vi "声音识别.vi"() -> ()   [LabVIEW 2014]
uses:
  <vilib>/sound/lvsound.llb/Sound Format.ctl
  <vilib>/Analysis/4window.llb/windowTd.ctl
  <vilib>/Analysis/1siggen.llb/Ramp Pattern by Samples.vi
  <vilib>/Analysis/NI_AALPro.lvlib
  <vilib>/Analysis/NI_AALBase.lvlib
panel:
  in  "停止":bool
  out "主频":i32
  in  "低频点":i32=90
  in  "高频点":i32=120
  out "模板2匹配":bool[](array[boolean])
  out "模板1匹配":bool[](array[boolean])
  in  "选项卡控件":enum32{"参数设置", "声卡设置"}(tab)
  in  "存模板1":bool caption="模板1"
  in  "存模板2":bool caption="模板2"
  in  "滤波器类型":i32(ring)=1 items=["低通", "高通", "带通", "带阻"]
  in  "高截止频率":dbl=2000.0 format="%.2f"
  in  "低截止频率":dbl=60.0 format="%.2f"
  in  "阶数":dbl=2.0 format="%.2f"
  in  "滤波器选择":u16(ring) items=["切比雪夫", "巴特沃斯", "无"]
  in  "截取声音长度":u16(ring)=512 items=["256"=256, "512"=512, "1024"=1024, "2048"=2048]
  in  "sound format":T1={"sound quality"=enum."mono", "rate"=enum."44100", "bits per sample"=enum."16 bit"} caption="声音格式"
  out "模板2":dbl[](array[numeric])=[-1.0, -0.9999784757638632, -0.999883730923308, -0.9997268308186364, -0.9996087454137307, -0.9995485640574947, -0.9996660148873113, -0.9996460865374096, -0.9990520630289842, -0.9996447767562398, -0.9988842018427372, -0.9988326168901588, -0.9994362746882363, -0.9994043225637047, -0.9996462893274354, -0.999250094691715, -0.9996529817000758, -0.9990974819147969, -0.9998535553541484, -0.9991407864070688, -0.9996794207758661, -0.9998567670842584, -0.9987714624308643, -0.9988979613875477, -0.9981546271077171, -0.99883165401242, -0.999806679939325, -0.9987834495902463, -0.9987170240934524, -0.9986010051790879, -0.9987859779624924, -0.99882513551929, -0.997846064915957, -0.9984471292033844, -0.9989846697345478, -0.9955902561514854, -0.9969375334942442, -0.9985341827269754, -0.9965219910541883, -0.997115233753815, -0.993177621304976, -0.9965369004229736, -0.996247289114047, -0.9965205723109544, -0.9929438024310587, -0.9921813234142332, -0.9923201356826735, -0.9902234197893732, -0.9875050624228046, -0.989978196297217, -0.9899613444021288, -0.9918200276943172, -0.9971748873436627, -0.9936090106840292, -0.9967077448120892, -0.99511317548537, -0.9900547089248353, -0.9915800418719736, -0.9951413205793777, -0.9983222383099732, -0.9983608025847126, -0.9943812759685029, -0.9907756695115925, -0.9910720617475026, -0.9942178283545733, -0.9960071684133079, -0.9947937292245801, -0.9894896646443787, -0.9936749087846007, -0.9986512039031801, -0.9924143125896042, -0.980352872634244, -0.9824158782190716, -0.9882635976611835, -0.9901615400254588, -0.9919879388627098, -0.9929695103692736, -0.9877372544473346, -0.9805321538200102, -0.9723162365341282, -0.9941849154146257, -0.9840418140212489, -0.9785614847877063, -0.9824280510357281, -0.9867776675701149, -0.989155265948291, -0.959160539004141, -0.9312115293907393, -0.924354536297946, -0.9169346034235589, -0.8821247424630705, -0.8638200718968311, -0.8820381048063836, -0.8904287781253226, -0.9186931656047802, -0.942467209539949, -0.9699323519669453, -0.9250753283046158, -0.8718873253555477, -0.8098010457230395, -0.6438727171847084, -0.5912443735241202, -0.7180949540210455, -0.7925349074727238, -0.8919213441425387, -0.8216144716655984, -0.5368039369940907, 0.38886068201338786, 1.0, 0.6065901128787996, -0.20578452524169594, -0.7248999522627186, -0.2749060806920392, 0.07040699283848677, 0.20626459396102206, -0.6102790238762816, -0.9134055836786642, -0.7114504523727746, -0.7787453756820504, -0.859195534470781, -0.6880456234367622, -0.7299328777920452, -0.8034112990123619, -0.7055433624855977, -0.6209224724888913, -0.6474430060007278, -0.6853656731838219, -0.7880905992092426, -0.7444394149310075, -0.9645654801987125, -0.7999452801476307, -0.752200101981826, -0.8948902768790076, -0.8933806119480991, -0.8823017299687642, -0.890886560515635, -0.8894321070807407, -0.8931547753090853, -0.9024438478576883, -0.9100495728196057, -0.911710889209407, -0.9445607561993957, -0.934249135253627, -0.904622091171806, -0.9145055185111371, -0.9628988334908968, -0.9810482464122726, -0.9675874443472068, -0.9621073803076765, -0.9713548954675296, -0.9660622852612207, -0.9439683935237438, -0.9418754698265419, -0.8686568800086364, -0.8092213616083905, -0.940425733399551, -0.9776850827528062, -0.8862970504440179, -0.9269686448441248, -0.9099397807879568, -0.871091321004459, -0.9251669503520498, -0.870146078274874, -0.8803470041783565, -0.6713148081403661, -0.5631453856847152, -0.7665886339386746, -0.9281502818635933, -0.8585161842069289, -0.8024715744018525, -0.8640915179082923, -0.982903824511303, -0.9084909144977602, -0.9722706899843834, -0.9511848674781466, -0.9756589379575122, -0.9787725658314163, -0.9779327416650971, -0.9439377043809586, -0.9291086359847139, -0.8921828883844908, -0.9143793651663683, -0.9233756179572645, -0.9185923843915021, -0.9318259983275918, -0.9312581662523354, -0.8123630832803784, -0.9058753941243535, -0.9432787247324338, -0.9211728624213069, -0.9207238178928795, -0.9020317894743983, -0.8030669530300928, -0.9149433950504898, -0.8616148769398828, -0.7970254148485149, -0.8422440070070124, -0.9125984117938313, -0.9666901859057956, -0.9554246868812509, -0.9894087763072112, -0.956459144652997, -0.9895936405317033, -0.9508371758791279, -0.9200188029869003, -0.9188388870802612, -0.9054584481957318, -0.9429600768930849, -0.9565453895181422, -0.912122419053691, -0.9518819229936425, -0.932683087820026, -0.9278028819493312, -0.9301165652301076, -0.9884957237600749, -0.963040376268851, -0.9655209194019106, -0.8980835146551925, -0.9071915985495637, -0.9562287296834957, -0.9291749404704612, -0.9502166274672502, -0.9843686847549361, -0.9582630331876297, -0.8514277714051874, -0.7171092057916761, -0.8531934139857488, -0.8057421106827759, -0.8013364169222371, -0.9706880418566048, -0.8994513795348863, -0.9430807290280687, -0.9803151690247353, -0.9414492030738784, -0.904749386470448, -0.8410294328838792, -0.8592362276422876, -0.8980549109925963, -0.9065637180637752, -0.9723695887006282, -0.8340799186010609, -0.8754020273712404, -0.940559734933539, -0.9521721965413019, -0.9548370301034873, -0.9603664110042679, -0.9433150050402023, -0.9925992527688022, -0.9720221075238545, -0.9797270980151095, -0.9706349822484007, -0.9919448347863793, -0.9852729642178658, -0.9949885259257842, -0.9770438736058363, -0.9700011832631854]
  out "模板1":dbl[](array[numeric])=[-0.9997440127807419, -0.9995220380571057, -0.9995902897348935, -0.9995357979586109, -0.9994879869517296, -0.9990814431600478, -0.999786870970356, -0.9991893733117945, -0.9998465713309023, -0.9998707870681628, -0.9999563774756277, -0.9983672987139602, -0.999880264902219, -0.9993717852254479, -0.9991030261051548, -0.9995136326835645, -0.9997645347029909, -0.9985313282076574, -0.9997301559393635, -0.9995234641757678, -0.9996431234057226, -0.999139315259616, -0.9995276217859526, -0.9991242785698715, -0.9991479330256554, -0.9992196130388197, -0.9978959279716081, -0.9995639207224252, -0.9985822974140731, -0.9960125349611552, -0.9980838017535006, -0.9964893672759322, -0.9946562731730431, -0.9969521384471256, -0.9959308295729385, -0.9957103403740175, -0.9966716950068587, -0.9969435987481197, -0.9967517577400672, -0.9934997828913328, -0.9952175081092053, -0.9984728596833808, -0.9983665702302467, -0.9953053980437071, -0.9899940068948201, -0.9927011727038199, -0.9974143037244904, -0.9920868374069218, -0.9915651780543104, -0.9946819848753914, -0.9902623232266299, -0.9923224250688908, -0.9962090994146557, -0.9974990188187914, -0.9987799073938248, -0.9964858261875376, -1.0, -0.9950122965483968, -0.9929111542282759, -0.99674771208652, -0.9954380057482245, -0.9960183527965598, -0.9932474770197688, -0.9924202965886824, -0.9937159036114802, -0.9961277720648933, -0.994216636633258, -0.9875978417778765, -0.9882092513484788, -0.9949915495928041, -0.9955829244113924, -0.9901426248726466, -0.991395073975417, -0.9905953370201996, -0.9911514283258394, -0.987816250459096, -0.9842971392499601, -0.9995689020137094, -0.9864129302652389, -0.9761006580004669, -0.9743217395433118, -0.9898417480030186, -0.9921504826964371, -0.9896286798607388, -0.994883499681581, -0.9917400884448188, -0.988557569471649, -0.9724526941106925, -0.9628869735613024, -0.9527110664883751, -0.9346277969487784, -0.9212021147305007, -0.9375774793281554, -0.9010715267204353, -0.9041357771905842, -0.8378382298396584, -0.7858040797157627, -0.7223403580528125, -0.7691362138013547, -0.7071423846830397, -0.7366525643253952, -0.5967453112567175, -0.3180470631746267, -0.5076573756976305, -0.7196194756151828, -0.08186718064963106, 0.7961248971775478, 1.0, 0.5552112778907459, 0.3990253476240408, 0.5109080507654662, -0.2785735567079543, -0.7506620703243985, -0.4927817111232846, -0.483965905877206, -0.6041468056765368, -0.5838158274395812, -0.6299950724589751, -0.4515955837929884, -0.3473300246823494, -0.27493629409090126, -0.3778189439187687, -0.9047044788114939, -0.9125457319727901, -0.6917499664860958, -0.820908917978653, -0.7887351137500261, -0.6863171530630592, -0.7540389449956904, -0.8954194739646075, -0.9797949126053243, -0.9391926191099735, -0.9617518755458666, -0.9769028522163401, -0.981834267740373, -0.9879277802829208, -0.9690035913867183, -0.9075597526810585, -0.9131141679460301, -0.9689403590135897, -0.9518375539572692, -0.932418020954141, -0.9907345002818224, -0.9352151553610134, -0.9754042431198124, -0.9744792471382142, -0.9135034124222947, -0.88790604896512, -0.8953500051967686, -0.8424796894419155, -0.8632615920880841, -0.9144833484778304, -0.989705625372779, -0.9284472966376549, -0.891815698550329, -0.9478387928405076, -0.9617910076411145, -0.9497526684178446, -0.9324675642722114, -0.9318933334867147, -0.9181840523695389, -0.8311457125542839, -0.7676439841445372, -0.8005356410093653, -0.8570505337551886, -0.6827327741635795, -0.6498853161064138, -0.8620072820776488, -0.8852296128964398, -0.916033416955761, -0.8949397345369553, -0.9851861839220112, -0.9666197661067494, -0.9594296686550134, -0.9167209070151537, -0.9505919554506888, -0.9657605440551648, -0.9694019401743963, -0.9588227257634793, -0.975917187129433, -0.9941311609332887, -0.9433572917808783, -0.905603106608587, -0.8562038779918986, -0.8795319913680256, -0.9335791148555251, -0.9105308626129569, -0.9402508260987222, -0.8899668077543964, -0.8470648184086745, -0.8301541884713339, -0.9202060587012243, -0.9291110562985246, -0.9261714239984843, -0.8587286529637863, -0.8723476053091272, -0.9071398954622749, -0.828077794521284, -0.8818237777512118, -0.8778091791269944, -0.9038464385525818, -0.9466723838674097, -0.9499470992199203, -0.9562232197422296, -0.9614154882608102, -0.958781143030921, -0.9867981001133651, -0.9166251404729362, -0.9359395991956431, -0.9523477739081351, -0.9500664215791567, -0.9550812963994444, -0.9798409351411519, -0.9564507980032216, -0.9729768220978592, -0.970004723139876, -0.9209757337818635, -0.8770281983081171, -0.8767785407913794, -0.9117690657496551, -0.9346202278845188, -0.8375077283102528, -0.8180037177118068, -0.7797125386786056, -0.8573786218023991, -0.965206732009058, -0.8696380239589367, -0.9043152036505393, -0.869985486830256, -0.8880174678215673, -0.9076883100998964, -0.9504304855590684, -0.9911949233816992, -0.9568545083751834, -0.9254572654577123, -0.9209456771528315, -0.9534217794961622, -0.9664337083514177, -0.9635839136536124, -0.9314469505325932, -0.9229998112610136, -0.9708121796305168, -0.9122730496181972, -0.9274734699377137, -0.9226054669470258, -0.9374491149297223, -0.9725365734899619, -0.9252092463239182, -0.9590977835663897, -0.9555009451185412, -0.9652718417072434, -0.9753048479679207, -0.9741915572832848, -0.9752978854562108, -0.9818650401740803, -0.9913380917200983]
  out "FFT输出":dbl[][](graph)
  out "截取声音":dbl[](graph) caption="单声道16位"
  in  "触发线":dbl(slide)=6064.2281879194625 caption="滑动杆" scale=30.0..30000.0
  out "滤波结果":dbl[][](graph) caption="单声道16位"
  # "基于声卡的语音识别系统"
  # "调节红线触发信号"
  # "鼠标进入录制样板\n鼠标离开结束"
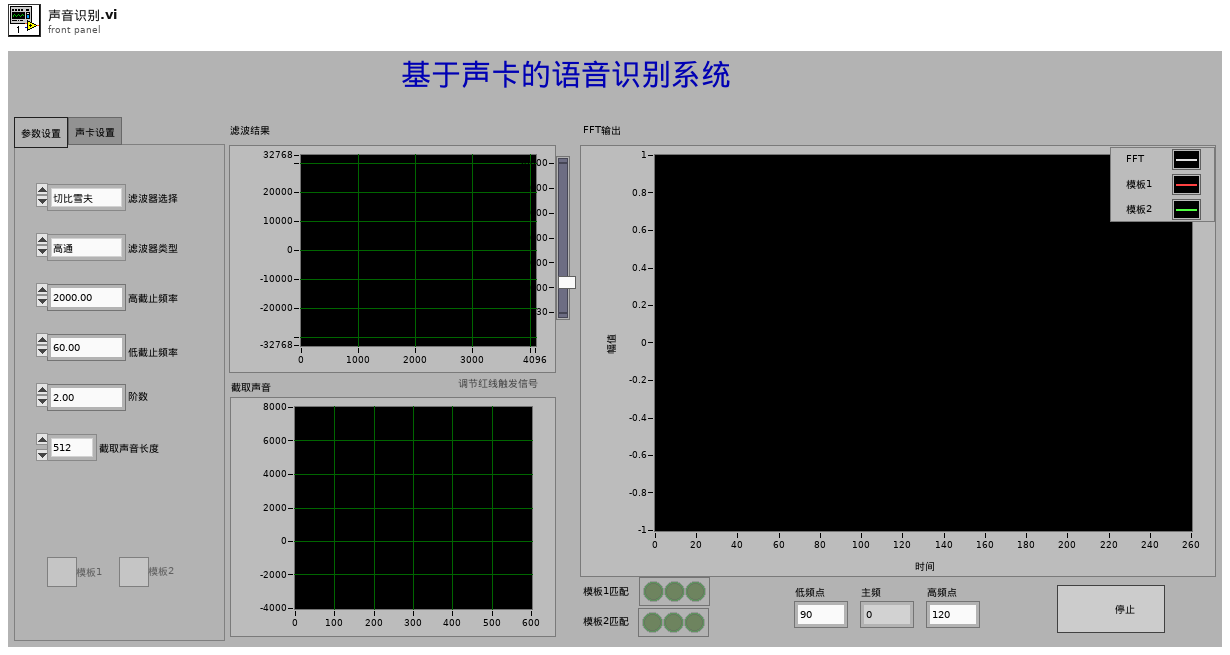
[diagram p1: front panel]
types:
  T1 = typedef "Sound Format.ctl" = cluster{"sound quality":enum16{"mono", "stereo"}, "rate":enum16{"11025", "22050", "44100", "8000"}, "bits per sample":enum16{"8 bit", "16 bit"}}
  T2 = typedef "NI_AALPro.lvlib/windowTd.ctl" = u32
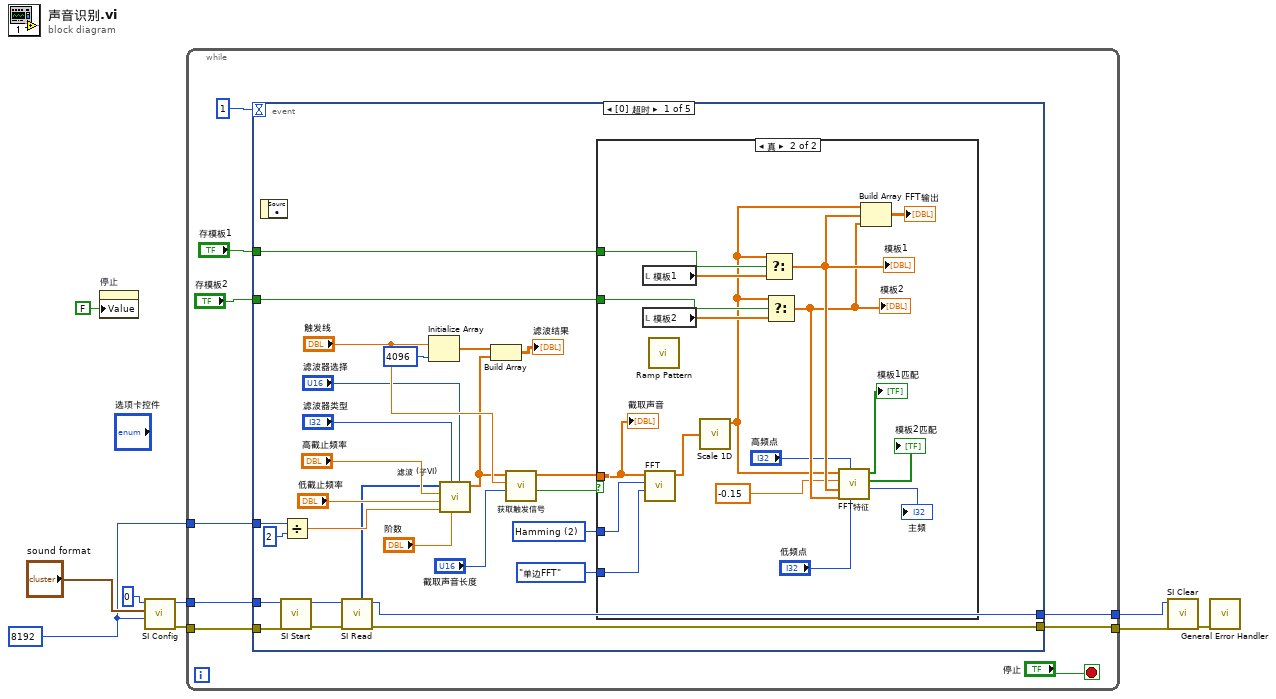
[diagram p0: block diagram]
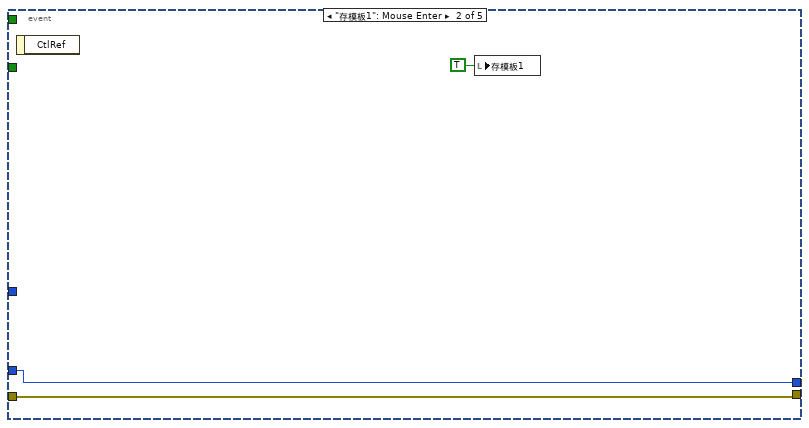
[diagram p3: hidden frame]
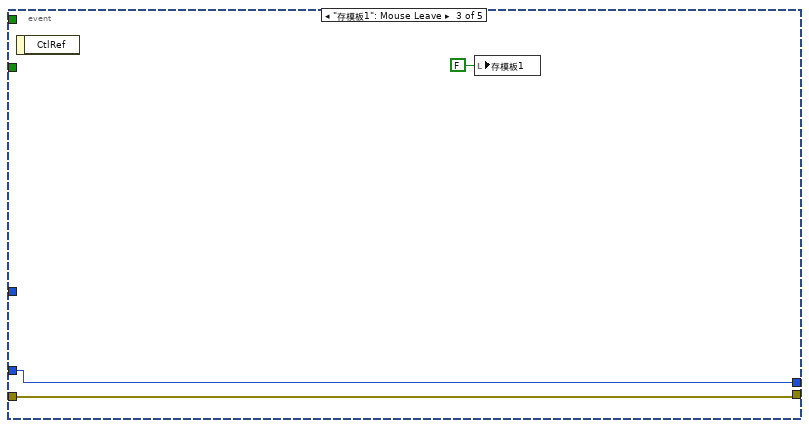
[diagram p4: hidden frame]
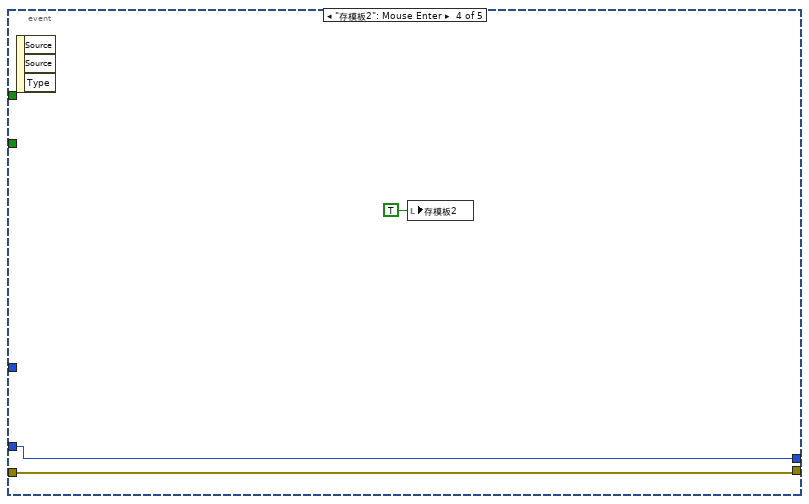
[diagram p5: hidden frame]
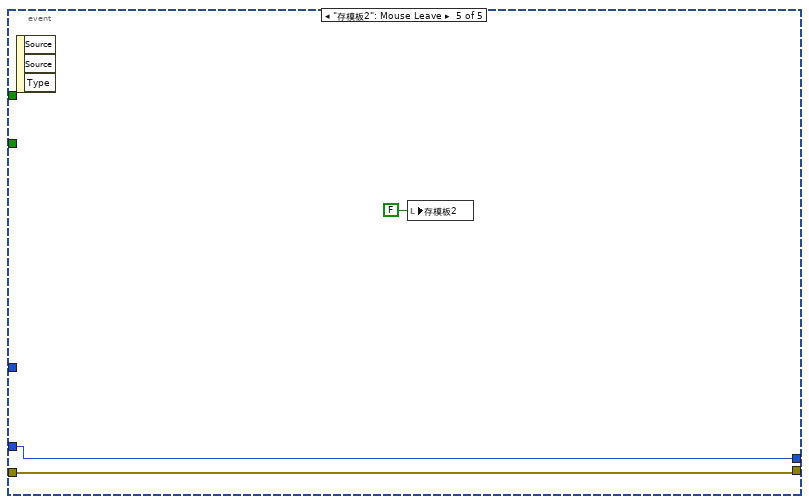
[diagram p6: hidden frame]
diagram:
  w2 = u32 8192 ("缓存")
  n1 = property on="停止" class="Bool (严格)"("Value"=FALSE ("停止")) -> ()  [unwired: 2 in, 2 out]
  n2 = call <vilib>:"SI Config.vi"("buffer size (8192 in bytes)"=w2, "sound format"="sound format", "device (0)"=u32 0 ("device")) -> ("error out"=w6:errorcluster, "task ID out"=w8:u32)  [unwired: 7 in]
  n3 = while {
    tunnel: w8 -> [w18]
    tunnel: [w17] -> w7
    tunnel: w2 -> [w13]
    tunnel: w6 -> [w16]
    tunnel: [w15] -> w5
    stop <- "停止" stop-if-true
    n4 = event shown="[0] 超时" {
      selector: _ -> [_ _ _ _ _]
      dyn-events: _ -> [_ _ _ _ _]
      timeout: 1 -> [_ _ _ _ _]
      tunnel: w18 -> [w43 w66 w69 w72 w75]
      tunnel: [w42 w66 w69 w72 w75] -> w17
      tunnel: w16 -> [w41 w65 w68 w71 w74]
      tunnel: [w40 w65 w68 w71 w74] -> w15
      tunnel: w13 -> [w30 _ _ _ _]
      tunnel: "存模板2" -> [w22 _ _ _ _]
      tunnel: "存模板1" -> [w21 _ _ _ _]
      event Timeout {
        w24 = T2 2 items=["矩形"=0, "Hanning"=1, "Hamming"=2, "Blackman-Harris"=3, "Exact Blackman"=4, "Blackman"=5, "Flat Top"=6, "4阶Blackman-Harris "=7, "7阶Blackman-Harris"=8, "Low Sidelobe"=9, "Blackman Nuttall"=11, "三角"=30, "Bartlett-Hanning"=31, "Bohman"=32, "Parzen"=33, "Welch"=34, "Kaiser"=60, "Dolph-Chebyshev"=61, "高斯"=62] ("window")
        n5 = event-data() -> ()  [unwired: 1 in, 1 out]
        n6 = call <vilib>:"SI Start.vi"("error in (no error)"=w41, "task ID in"=w43) -> ("error out"=w44:errorcluster, "task ID out"=w45:u32)  [unwired: 8 in]
        n7 = Divide(x=w30, y=u32 2) -> (x/y=w28:dbl)
        n8 = call <vilib>:"SI Read.vi"("error in (no error)"=w44, "task ID in"=w45) -> ("error out"=w40:errorcluster, "task ID out"=w42:u32, "mono 16-bit"=w19:i16[])  [unwired: 4 in, 3 out]
        n9 = Initialize Array("触发线", 4096 ("维数大小")) -> (w37:dbl[])
        n10 = call "滤波 (子VI).vi"("滤波器选择"="滤波器选择", "阶数"="阶数", "滤波器类型"="滤波器类型", "采样率"=w28, "低截止频率"="低截止频率", "高截止频率"="高截止频率", "X输入"=w19) -> ("滤波输出"=w36:dbl[])  [unwired: 4 in]
        n11 = Build Array(w37, w36) -> (→"滤波结果":dbl[][])
        n12 = call "获取触发信号.vi"("截取信号长度"="截取声音长度", "触发"="触发线", "输入信号"=w36) -> ("触发"=w26:bool, "截取信号"=w20:dbl[])  [unwired: 7 in]
        n13 = case shown="真" w26 {
          tunnel: w24 -> [_ w62]
          tunnel: enum16{"对称FFT", "单边FFT", "FFT功率"}."单边FFT" ("FFT模式") -> [_ w61]
          tunnel: w22 -> [_ w58]
          tunnel: w21 -> [_ w57]
          tunnel: w20 -> [_ w54]
          frame False {
          }
          frame True {
            n14 = local read "模板1"() -> (w55:dbl[])
            n15 = local read "模板2"() -> (w56:dbl[])
            n16 = call "FFT.vi"("FFT模式"=w61, "window"=w62, "输入X"=w54) -> ("FFT输出"=w53:dbl[])  [unwired: 8 in]
            n17 = call-poly <vilib>:"Ramp Pattern.vi"() -> ()  [unwired: 10 in, 2 out]
            n18 = call <vilib>:"Scale 1D.vi"("X"=w53) -> ("Y=(X-offset)/scale"=w52:dbl[])  [unwired: 3 out]
            n19 = Select(t=w52, s=w57, f=w55) -> (s? t:f=w60:dbl[])
            "模板1" <- w60
            n20 = Select(t=w52, s=w58, f=w56) -> (s? t:f=w59:dbl[])
            "模板2" <- w59
            n21 = call "FFT特征.vi"("低频点"="低频点", "高频点"="高频点", "样板2"=w59, "样板"=w60, "幅度误差"=-0.15, "输入"=w52) -> ("主频"=→"主频":i32, "样板2匹配"=→"模板2匹配":bool[], "样板1匹配"=→"模板1匹配":bool[])  [unwired: 3 in]
            n22 = Build Array(w52, w60, w59) -> (→"FFT输出":dbl[][])
            "截取声音" <- w54
          }
        }
      }
      event "存模板1": Mouse Enter {
        n23 = event-data() -> ()  [unwired: 1 in, 1 out]
        n24 = local write "存模板1"(TRUE ("存模板1")) -> ()
      }
      event "存模板1": Mouse Leave {
        n25 = event-data() -> ()  [unwired: 1 in, 1 out]
        n26 = local write "存模板1"(FALSE ("存模板1")) -> ()
      }
      event "存模板2": Mouse Enter {
        n27 = event-data() -> ()  [unwired: 1 in, 3 out]
        n28 = local write "存模板2"(TRUE ("存模板2")) -> ()
      }
      event "存模板2": Mouse Leave {
        n29 = event-data() -> ()  [unwired: 1 in, 3 out]
        n30 = local write "存模板2"(FALSE ("存模板2")) -> ()
      }
    }
  }
  n31 = call <vilib>:"SI Clear.vi"("error in (no error)"=w5, "task ID in"=w7) -> ("error out"=w4:errorcluster)  [unwired: 9 in]
  n32 = call <vilib>:"General Error Handler.vi"("error in (no error)"=w4) -> ()  [unwired: 10 in, 5 out]
